vi "SerialPoll ConvBox.vi"(8 "error in":errorcluster, 10 "address string":string, 11 "VISA resource in":refnum<visa-resource-name>) -> (0 "error out":errorcluster, 1 "ibsta":T1, 2 "serial poll byte":i16, 3 "VISA resource out":refnum<visa-resource-name>)   [LabVIEW 2023, in "Protocols.lvlib" / "RS-xxx to GPIB ConvBox.lvclass"]
uses:
  RS-xxx to GPIB ConvBox.lvclass
  <vilib>/Instr/_visa.llb/GPIB Status Boolean Array.ctl
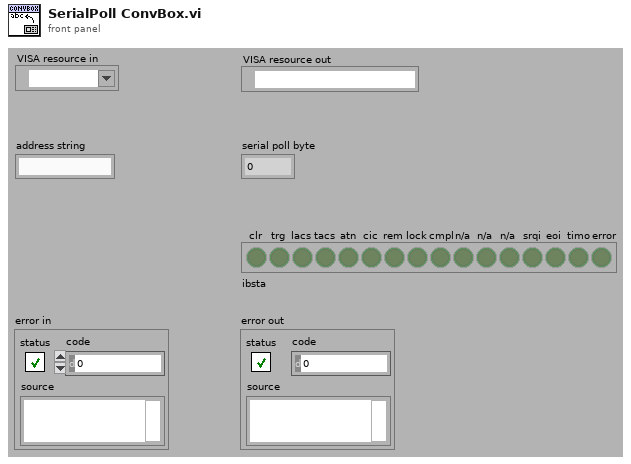
[diagram p1: front panel]
types:
  T1 = typedef "GPIB Status Boolean Array.ctl" = bool[]
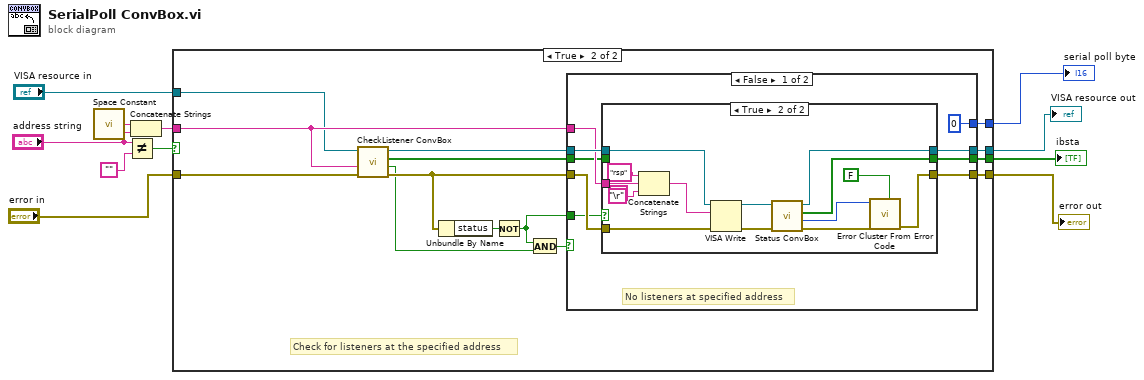
[diagram p0: block diagram]
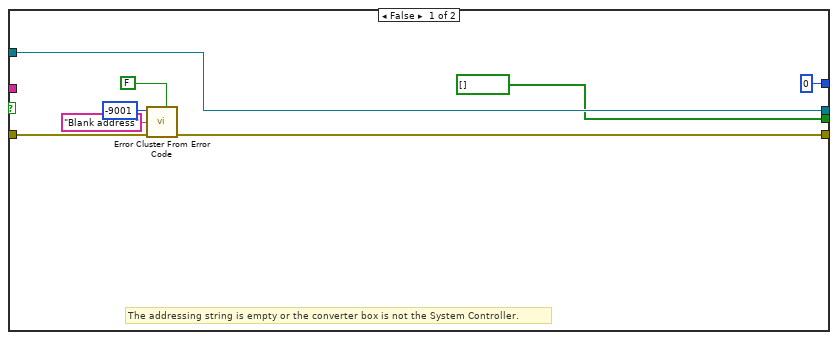
[diagram p2: hidden frame]
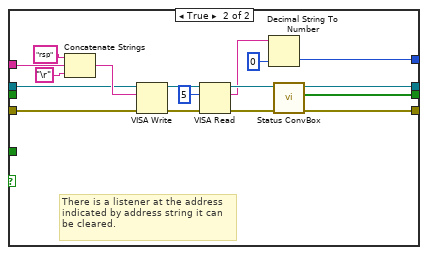
[diagram p4: hidden frame]
diagram:
  n1 = call <vilib>:"Space Constant.vi"() -> ("String"=w8:string)
  n2 = Not Equal?(x="address string", y="") -> (x != y?=w10:bool)
  n3 = Concatenate Strings(w8, "address string") -> (w5:string)
  n4 = case shown="True" w10 {
    tunnel: [w19 w33] -> w4
    tunnel: [T1 [] ("ibsta") w32] -> w2
    tunnel: [w16 w31] -> w3
    tunnel: w5 -> [_ w28]
    tunnel: "error in" -> [w17 w30]
    tunnel: "VISA resource in" -> [w19 w27]
    tunnel: [i16 0 w20] -> w1
    frame False {
      # "The addressing string is empty or the converter box is not the System Controller."
      n5 = call <vilib>:"Error Cluster From Error Code.vi"("is warning? (False)"=FALSE, "error in (no error)"=w17, "error message (\"\")"="Blank address" ("error message (\"\")"), "error code (0)"=-9001) -> ("error out"=w16:errorcluster)  [unwired: 5 in]
    }
    frame True {
      # "Check for listeners at the specified address"
      n6 = call "CheckListener ConvBox.vi"("error in"=w30, "address string"=w28, "VISA resource in"=w27) -> ("error out"=w26:errorcluster, "listener found"=w24:bool, "ibsta"=w22:T1, "VISA resource out"=w29:refnum<visa-resource-name>)  [unwired: 5 in]
      n7 = Unbundle By Name(w26) -> ("status"=w23:bool)
      n8 = Not(x=w23) -> (.not. x?=w21:bool)
      n9 = And(x=w21, y=w24) -> (x .and. y?=w25:bool)
      n10 = case shown="False" w25 {
        tunnel: [w39 w76] -> w33
        tunnel: [w38 w75] -> w32
        tunnel: [w42 w74] -> w31
        tunnel: w26 -> [w41 w73]
        tunnel: w29 -> [w40 w69]
        tunnel: w28 -> [w37 w68]
        tunnel: w22 -> [w35 _]
        tunnel: w21 -> [w36 _]
        tunnel: [i16 0 w60] -> w20
        frame False {
          (unwired) "\r"
          # "No listeners at specified address"
          n11 = case shown="True" w36 {
            tunnel: [w43 w58] -> w42
            tunnel: w41 -> [w43 w55]
            tunnel: w40 -> [w44 w53]
            tunnel: [w44 w52] -> w39
            tunnel: [w45 w50] -> w38
            tunnel: w37 -> [_ w49]
            tunnel: w35 -> [w45 _]
            frame False {
              # "Error found in checklistener"
            }
            frame True {
              n12 = Concatenate Strings("rsp", w49, "\r") -> (w56:string)
              n13 = VISA Write(VISA resource name=w53, write buffer=w56, error in (no error)=w55) -> (VISA resource name out=w47:refnum<visa-resource-name>, error out=w46:errorcluster)  [unwired: 1 out]
              n14 = call "Status ConvBox.vi"("error in (no error)"=w46, "VISA resource name"=w47) -> ("error out"=w54:errorcluster, "GPIB error"=w51:i16, "ibsta"=w50:T1, "VISA resource out"=w52:refnum<visa-resource-name>)  [unwired: 6 in]
              n15 = call <vilib>:"Error Cluster From Error Code.vi"("is warning? (False)"=FALSE, "error in (no error)"=w54, "error code (0)"=w51) -> ("error out"=w58:errorcluster)  [unwired: 6 in]
            }
          }
        }
        frame True {
          # "There is a listener at the address\nindicated by address string it can\nbe cleared."
          n16 = Concatenate Strings("rsp", w68, "\r") -> (w70:string)
          n17 = VISA Write(VISA resource name=w69, write buffer=w70, error in (no error)=w73) -> (VISA resource name out=w66:refnum<visa-resource-name>, error out=w64:errorcluster)  [unwired: 1 out]
          n18 = VISA Read(VISA resource name=w66, byte count=u32 5, error in (no error)=w64) -> (VISA resource name out=w65:refnum<visa-resource-name>, read buffer=w62:string, error out=w63:errorcluster)  [unwired: 1 out]
          n19 = Decimal String To Number(string=w62, default (0L)=i16 0 ("default (0 I32)")) -> (number=w60:i16)  [unwired: 1 in, 1 out]
          n20 = call "Status ConvBox.vi"("error in (no error)"=w63, "VISA resource name"=w65) -> ("error out"=w74:errorcluster, "ibsta"=w75:T1, "VISA resource out"=w76:refnum<visa-resource-name>)  [unwired: 6 in, 1 out]
        }
      }
    }
  }
  "serial poll byte" <- w1
  "VISA resource out" <- w4
  "ibsta" <- w2
  "error out" <- w3
